vi "Ordre 1.vi"(11 "Tableau":dbl[](array[numeric])) -> (3 "Numérique":dbl format="%#_13g")   [LabVIEW 2018]
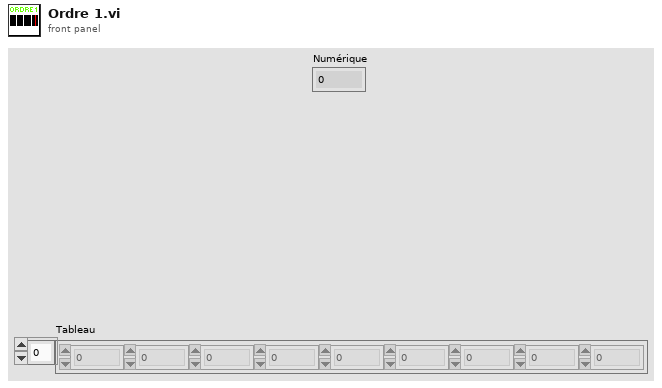
[diagram p1: front panel]
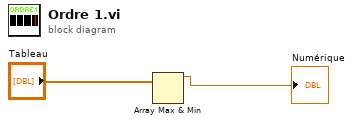
[diagram p0: block diagram]
diagram:
  n1 = Array Max & Min(array="Tableau") -> (max value=→"Numérique":dbl)  [unwired: 3 out]
